vi "GetReference.vi"(8 "error in (no error)":errorcluster, 10 "Label":string, 11 "Framework Templates":refnum<vi>) -> (0 "error out":errorcluster, 2 "Scrollbar":refnum<vi>, 3 "Graphic":refnum<vi>)   [LabVIEW 2020, in "FakedArray.lvclass"]
uses:
  FakedArray.lvclass
  vi.lib/LabVIEW Icon API/lv_icon/Controls/Graphic.ctl
panel:
  in  "Scrollbar":refnum<vi>
  in  "Graphic":refnum<vi>
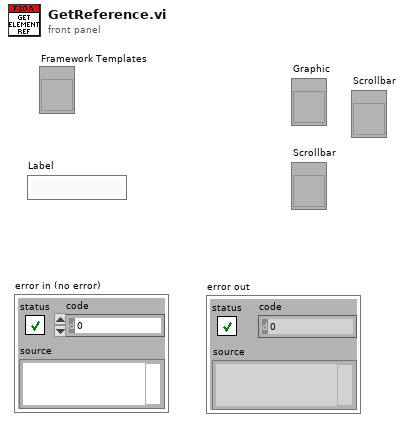
[diagram p1: front panel]
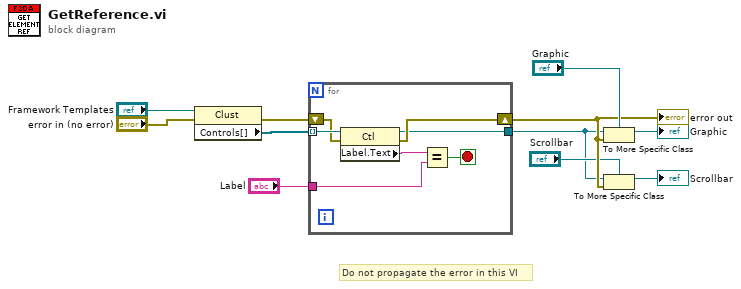
[diagram p0: block diagram]
diagram:
  # "Do not propagate the error in this VI"
  n1 = property class="Clust"(reference="Framework Templates", error in="error in (no error)") -> (error out=w10:errorcluster, "Controls[]"=w8:refnum<vi>[])  [unwired: 1 out]
  n2 = for {
    shift-right: [w13] -> w6
    shift-left: w10 -> [w14]
    tunnel: "Label" -> [w16]
    tunnel: w8 -> [w18] mode=indexing
    tunnel: [w12] -> w2
    stop <- w15 stop-if-true
    n3 = property class="Ctl"(reference=w18, error in=w14) -> (reference out=w12:refnum<vi>, error out=w13:errorcluster, "Label.Text"=w17:string)
    n4 = Equal?(x=w17, y=w16) -> (x = y?=w15:bool)
  }
  "error out" <- w6
  n5 = To More Specific Class(target class="Graphic", reference=w2, error in=w6) -> (specific class reference=→"Graphic":refnum<vi>)  [unwired: 1 out]
  n6 = To More Specific Class(target class="Scrollbar", reference=w2, error in=w6) -> (specific class reference=→"Scrollbar":refnum<vi>)  [unwired: 1 out]
